vi "SlaveAccelerometerSample3.vi"   [LabVIEW 2016]
uses:
  <vilib>/rvi/Emulation/niFpgaGetClockAttributes.vi
  <vilib>/rvi/Emulation/niFpgaSctlEmulationGetInTimedLoop.vi
  <vilib>/rvi/Emulation/niFpgaEmulationReportErrorSimple.vi
  <vilib>/rvi/eio/common/nirviEmuTemplateMethod_errors.vi
  <vilib>/rvi/Emulation/niFpgaEmulationIsFPGAContextNoSignature.vi
  <vilib>/rvi/DataTransferAndStorage/Container/Common/niFpgaContainerGetUniqueNameForEmu.vi
  <vilib>/rvi/Memory/Memory_Emulation/niFpgaMemoryEmulationCacheClearOnFirstRun.vi
  <vilib>/rvi/Memory/Memory_Emulation/nirvimemoryEmulationManagerCache_MakeExclusive.vi
  <vilib>/rvi/Memory/Memory_Emulation/niFpgaMemoryEmulationValidateCache.vi
  <vilib>/rvi/Memory/Memory_Emulation/nirvimemoryEmulationManagerCache_InsertValue.vi
  <vilib>/Utility/error.llb/Clear Errors.vi
  <vilib>/rvi/Memory/Memory_Emulation/nirvimemoryEmulationManagerCache_ReleaseExclusive.vi
  <vilib>/rvi/Memory/Memory_Emulation/nirvimemoryEmulationManagerCache_GetValue.vi
  <vilib>/rvi/Memory/Memory_Emulation/nirvimemoryEmulationManagerCache_SetValue.vi
  <vilib>/rvi/Emulation/niFpgaProcessEmulError.vi
  <vilib>/rvi/errors/niFpgaSetErrorForExecOnDevCompSimple.vi
  <vilib>/rvi/eio/common/nirviEmuReportErrorAndStop.vi
  <vilib>/rvi/FIFO/Fifo_Resource/nirvififoEmulationSetSize.vi
  <vilib>/rvi/FIFO/Fifo_Resource/nirviFifoEmulationQueueMgr.vi
  <instcachedir>/0/nirviFifoEmulationQueueMgr_E5CAEC123FF24DC58D834DCA3CDAA9B5.lvgen/nirviFifoEmulationQueueMgr_E5CAEC123FF24DC58D834DCA3CDAA9B5_007.vi
  <vilib>/rvi/FIFO/Fifo_Resource/nirvififoEmulationDetermineInputValidOut.vi
  <vilib>/rvi/FIFO/Fifo_Resource/nirvififoEmulationCreateLock.vi
  <vilib>/rvi/FIFO/Fifo_Resource/nirvififoEmulationObtainLock.vi
  <vilib>/rvi/FIFO/Fifo_Resource/nirvififoEmulationReleaseLock.vi
  <vilib>/rvi/occurrence/nirviWaitOnOccurrenceBase.vi
  <vilib>/rvi/errors/nirviReportUnexpectedCaseInternalError.vi
  <vilib>/rvi/errors/nirviReportUnexpectedCaseInternalError (U32).vi
  <instcachedir>/0/nirviFifoEmulationQueueMgr_E5CAEC123FF24DC58D834DCA3CDAA9B5.lvgen/nirviFifoEmulationQueueMgr_E5CAEC123FF24DC58D834DCA3CDAA9B5_005.vi
  <vilib>/rvi/Emulation/niFpgaCriticalErrorInLSC.vi
  <vilib>/eio/EIOMethodNode/EIOMethodNode.xnode
  <vilib>/eio/EIONode/EIONode.xnode
  <vilib>/rvi/DataTransferAndStorage/Container/XNode/niFpgaContainer.xnode
  <vilib>/rvi/DataTransferAndStorage/Register/Emulation/niFpgaRegisterEmulation.vi
  <vilib>/rvi/FIFO/Fifo_Resource/nirvififoEmulationWrite.vi
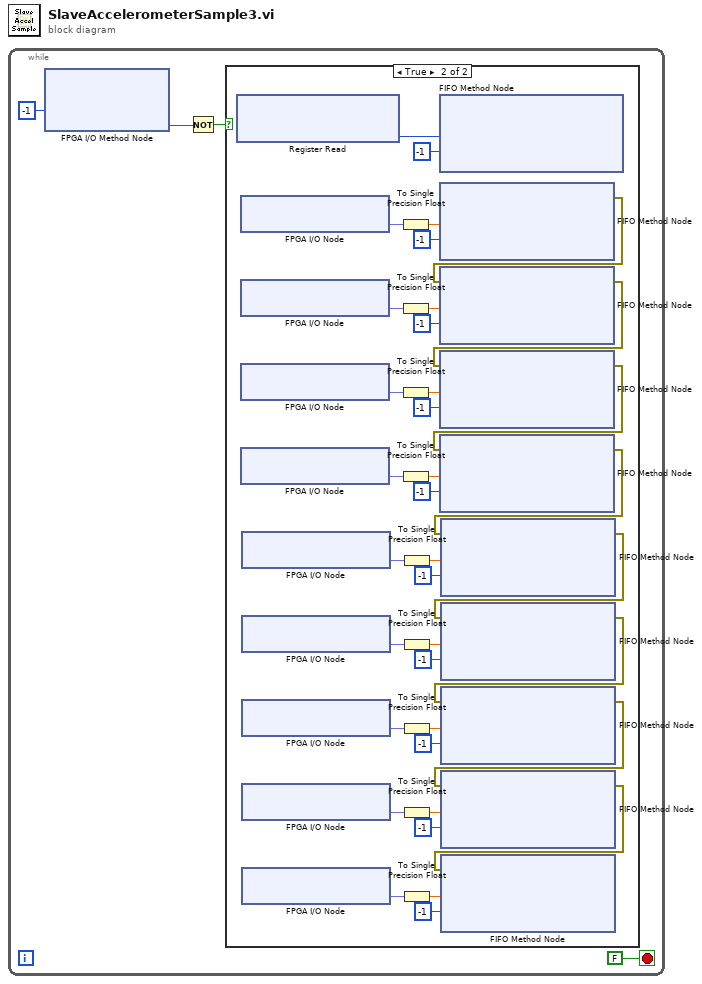
[diagram p0: block diagram]
diagram:
  n1 = while {
    stop <- FALSE stop-if-true
    n2 = xnode "FPGA I/O Method Node"("Timeout"=-1) -> ("Timed Out"=w3:bool)  [unwired: 1 in, 1 out]
    n3 = Not(x=w3) -> (.not. x?=w2:bool)
    n4 = case shown="True" w2 {
      frame False {
      }
      frame True {
        n5 = xnode "Register Read"() -> ("Data"=w5:u64)  [unwired: 1 in, 1 out]
        n6 = xnode "FPGA I/O Node"() -> ("Accelerometer1/AI0"=w40:fxp<+/-,24,7>)  [unwired: 1 in, 1 out]
        n7 = xnode "FPGA I/O Node"() -> ("Accelerometer1/AI1"=w35:fxp<+/-,24,7>)  [unwired: 1 in, 1 out]
        n8 = xnode "FPGA I/O Node"() -> ("Accelerometer1/AI2"=w27:fxp<+/-,24,7>)  [unwired: 1 in, 1 out]
        n9 = xnode "FPGA I/O Node"() -> ("Accelerometer2/AI0"=w32:fxp<+/-,24,7>)  [unwired: 1 in, 1 out]
        n10 = xnode "FPGA I/O Node"() -> ("Accelerometer2/AI1"=w11:fxp<+/-,24,7>)  [unwired: 1 in, 1 out]
        n11 = xnode "FPGA I/O Node"() -> ("Accelerometer2/AI2"=w16:fxp<+/-,24,7>)  [unwired: 1 in, 1 out]
        n12 = xnode "FPGA I/O Node"() -> ("Accelerometer3/AI0"=w24:fxp<+/-,24,7>)  [unwired: 1 in, 1 out]
        n13 = xnode "FPGA I/O Node"() -> ("Accelerometer3/AI1"=w19:fxp<+/-,24,7>)  [unwired: 1 in, 1 out]
        n14 = xnode "FPGA I/O Node"() -> ("Accelerometer3/AI2"=w7:fxp<+/-,24,7>)  [unwired: 1 in, 1 out]
        n15 = To Single Precision Float(number=w40) -> (single precision float=w39:sgl)
        n16 = To Single Precision Float(number=w35) -> (single precision float=w36:sgl)
        n17 = To Single Precision Float(number=w27) -> (single precision float=w28:sgl)
        n18 = To Single Precision Float(number=w32) -> (single precision float=w31:sgl)
        n19 = To Single Precision Float(number=w11) -> (single precision float=w12:sgl)
        n20 = To Single Precision Float(number=w16) -> (single precision float=w15:sgl)
        n21 = To Single Precision Float(number=w24) -> (single precision float=w23:sgl)
        n22 = To Single Precision Float(number=w19) -> (single precision float=w20:sgl)
        n23 = To Single Precision Float(number=w7) -> (single precision float=w8:sgl)
        n24 = xnode ("FIFO Method Node")("Element"=w5, "Timeout"=-1) -> ()  [unwired: 1 in, 2 out]
        n25 = xnode ("FIFO Method Node")("Element"=w39, "Timeout"=-1) -> ("error out"=w34:errorcluster)  [unwired: 2 in, 2 out]
        n26 = xnode ("FIFO Method Node")("Element"=w36, "Timeout"=-1, "error in (no error)"=w34) -> ("error out"=w26:errorcluster)  [unwired: 1 in, 2 out]
        n27 = xnode ("FIFO Method Node")("Element"=w28, "Timeout"=-1, "error in (no error)"=w26) -> ("error out"=w33:errorcluster)  [unwired: 1 in, 2 out]
        n28 = xnode ("FIFO Method Node")("Element"=w31, "Timeout"=-1, "error in (no error)"=w33) -> ("error out"=w10:errorcluster)  [unwired: 1 in, 2 out]
        n29 = xnode ("FIFO Method Node")("Element"=w12, "Timeout"=-1, "error in (no error)"=w10) -> ("error out"=w17:errorcluster)  [unwired: 1 in, 2 out]
        n30 = xnode ("FIFO Method Node")("Element"=w15, "Timeout"=-1, "error in (no error)"=w17) -> ("error out"=w25:errorcluster)  [unwired: 1 in, 2 out]
        n31 = xnode ("FIFO Method Node")("Element"=w23, "Timeout"=-1, "error in (no error)"=w25) -> ("error out"=w18:errorcluster)  [unwired: 1 in, 2 out]
        n32 = xnode ("FIFO Method Node")("Element"=w20, "Timeout"=-1, "error in (no error)"=w18) -> ("error out"=w6:errorcluster)  [unwired: 1 in, 2 out]
        n33 = xnode ("FIFO Method Node")("Element"=w8, "Timeout"=-1, "error in (no error)"=w6) -> ()  [unwired: 1 in, 3 out]
      }
    }
  }
